vi "Close Transport.vi"(8 "error in (no error)":errorcluster, 11 "ITransport in":refnum<class "ITransport.lvclass">) -> (0 "error out":errorcluster)   [LabVIEW 2017, in "IMediator.lvlib" / "ITransport.lvclass"]
uses:
  ITransport.lvclass
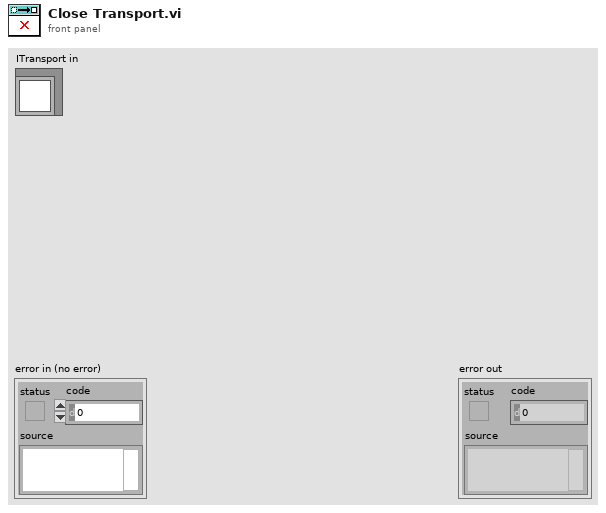
[diagram p1: front panel]
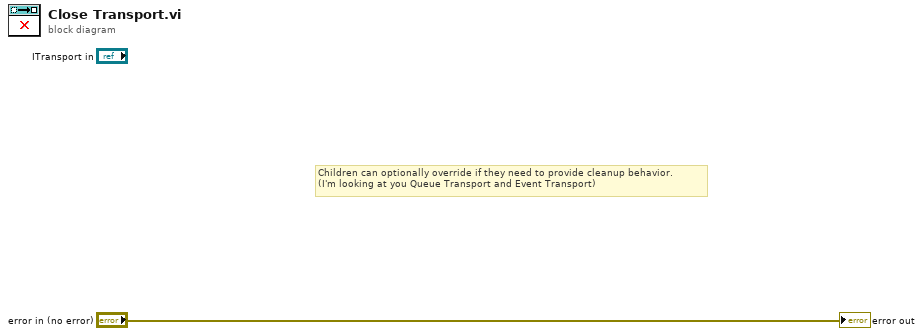
[diagram p0: block diagram]
diagram:
  # "Children can optionally override if they need to provide cleanup behavior.\n(I'm looking at you Queue Transport and Event Transport)"
  "error out" <- "error in (no error)"
